vi "OpenCamera.vi"(0 "object in":refnum<class "Hamamatsu.lvclass">, 5 "error in (no error)":errorcluster) -> (14 "object out":refnum<class "Hamamatsu.lvclass">, 15 "Sub Region":T2 {"V Size"."Value" min=0 max=0 step=4; "H Size"."Value" min=0 max=0 step=4; "V Offset"."Value" min=0 max=0 step=4; "H Offset"."Value" min=0 max=0 step=4}, 16 "CameraConnected":bool, 19 "error out":errorcluster)   [LabVIEW 2021, in "Hamamatsu.lvclass"]
uses:
  Hamamatsu.lvclass
  Hamamatsu.lvclass/Hamamatsu.ctl
  <vilib>/Utility/miscctls.llb/LVMinMaxIncTypeDef.ctl
panel:
  out "Camera Details":T3
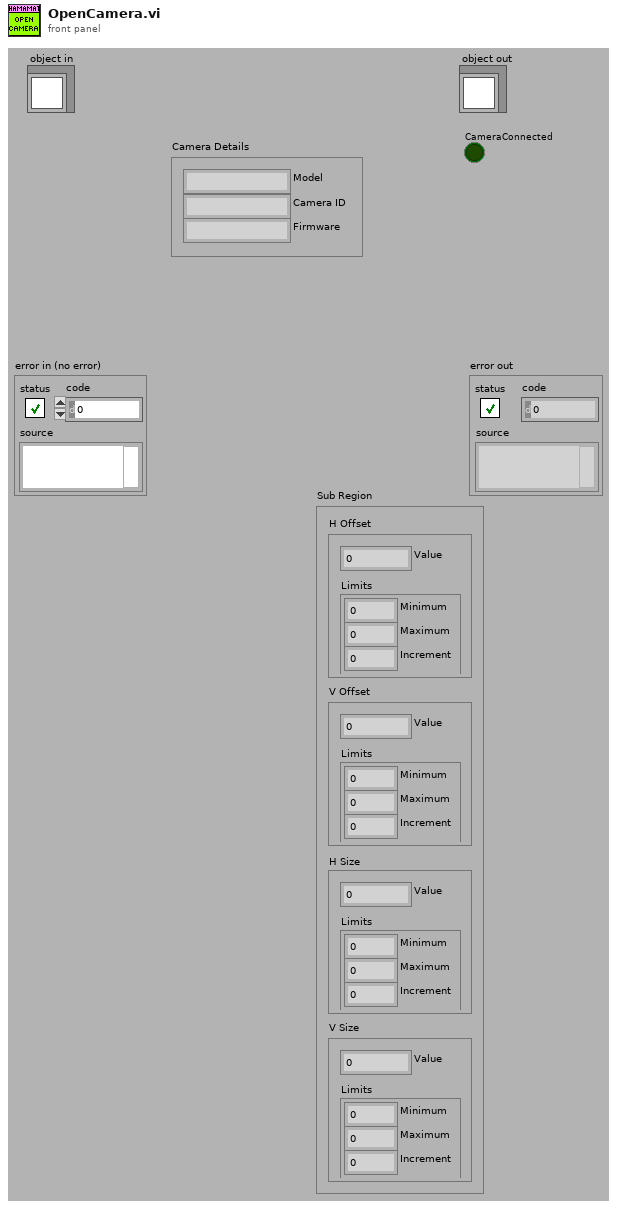
[diagram p1: front panel]
types:
  T1 = typedef "LVMinMaxIncTypeDef.ctl" = cluster{"Minimum":dbl, "Maximum":dbl, "Increment":dbl}
  T2 = cluster{"H Offset":cluster{"Value":i32, "Limits":T1}, "V Offset":cluster{"Value":i32, "Limits":T1}, "H Size":cluster{"Value":i32, "Limits":T1}, "V Size":cluster{"Value":i32, "Limits":T1}}
  T3 = cluster{"Model":string, "Camera ID":string, "Firmware":string}
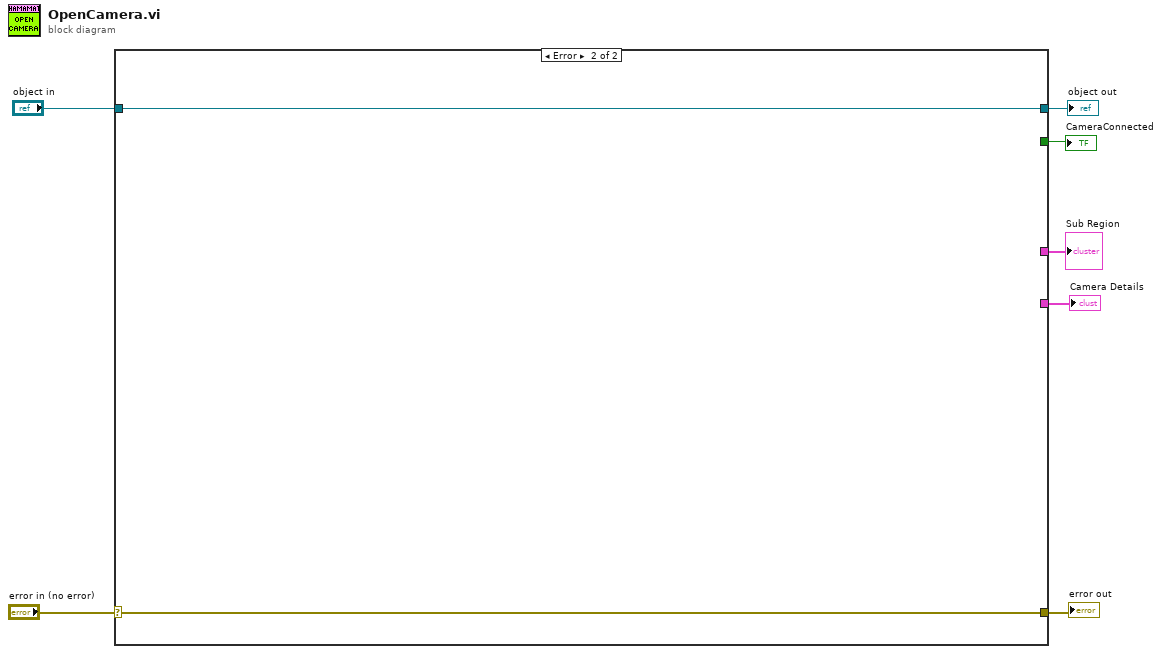
[diagram p0: block diagram]
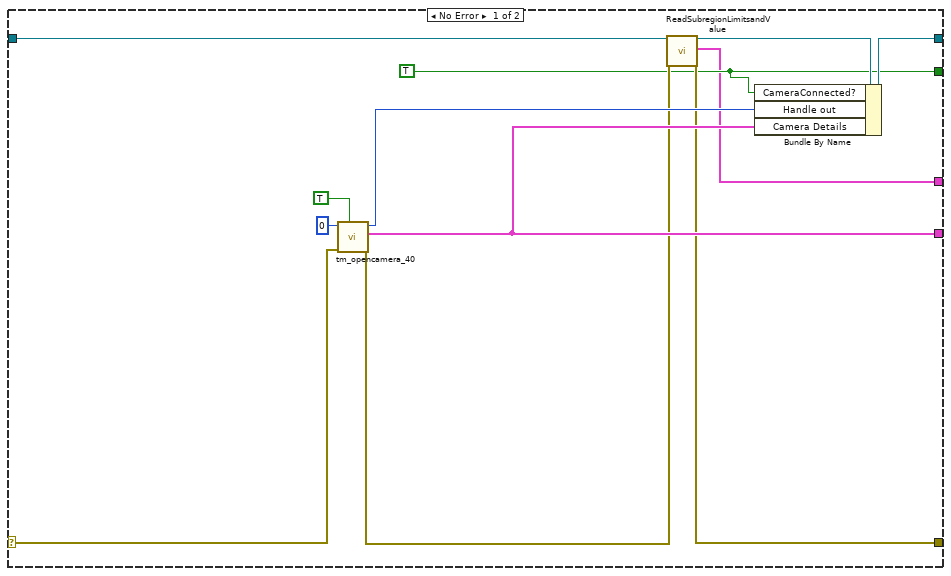
[diagram p2: hidden frame]
diagram:
  n1 = case shown="Error" "error in (no error)" {
    selector: "error in (no error)" -> [w16 w21]
    tunnel: [w12 w21] -> w6
    tunnel: [w18 w20] -> w4
    tunnel: "object in" -> [w13 w20]
    tunnel: [w17 _] -> w3
    tunnel: [w9 _] -> w2
    tunnel: [w8 _] -> w1
    frame No Error {
      w9 = TRUE ("CameraConnected")
      n2 = call <userlib>:"tm_opencamera_40.vi"("Force Open"=TRUE, "error in (no error)"=w16, "Camera Index"=u32 0) -> ("error out"=w14:errorcluster, "Camera Details"=w17:T3, "Handle out"=w15:u32)  [unwired: 6 in]
      n3 = call-dynamic "ReadSubregionLimitsandValue.vi"("object in"=w13, "error in (no error)"=w14) -> ("object out"=w11:refnum<class "Hamamatsu.lvclass">, "Sub Region"=w8:T2, "error out"=w12:errorcluster)  [unwired: 15 in]
      n4 = Bundle By Name(cluster=w11, "CameraConnected?"=w9, "Handle out"=w15, "Camera Details"=w17) -> (w18:refnum<class "Hamamatsu.lvclass">)
    }
    frame Error {
    }
  }
  "error out" <- w6
  "object out" <- w4
  "Camera Details" <- w3
  "CameraConnected" <- w2
  "Sub Region" <- w1
